vi "Read Database.vi"(8 "error in (no error)":errorcluster, 11 "Column Parent in":refnum<class "Column Parent.lvclass">) -> (0 "error out":errorcluster, 2 "Database":refnum<class "Database Interface.lvclass">, 3 "Column Parent out":refnum<class "Column Parent.lvclass">)   [LabVIEW 2020, in "Basic Columns.lvlib" / "Column Parent.lvclass"]
uses:
  Column Parent.lvclass
  Database Libraries/Database Interfaces/Database Interface Class/Database Interface.lvclass
  Column Interface/Column Configuration Interface Class/Column Configuration.lvclass
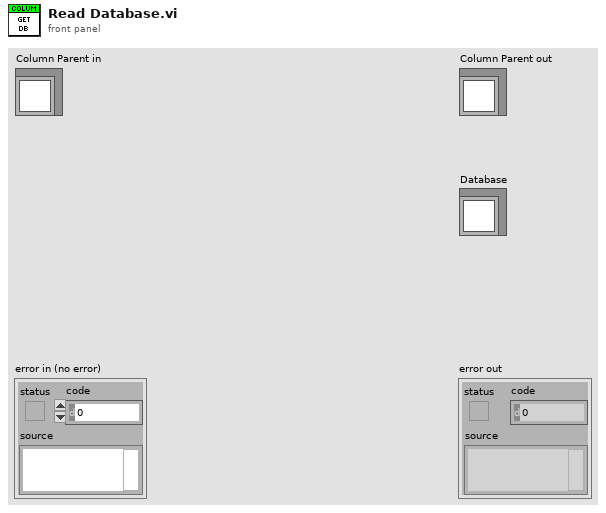
[diagram p1: front panel]
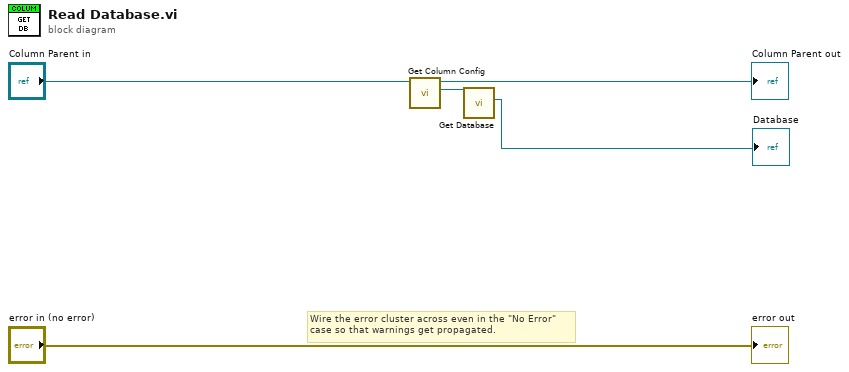
[diagram p0: block diagram]
diagram:
  # "Wire the error cluster across even in the \"No Error\"\ncase so that warnings get propagated."
  n1 = call-dynamic "Get Column Config.vi"("Column Parent in"="Column Parent in") -> ("Column Configuration"=w1:refnum<class "Column Configuration.lvclass">, "Column Parent out"=→"Column Parent out":refnum<class "Column Parent.lvclass">)  [unwired: 8 in, 1 out]
  n2 = call-dynamic "Get Database.vi"("Column Configuration in"=w1) -> ("Database"=→"Database":refnum<class "Database Interface.lvclass">)  [unwired: 8 in, 2 out]
  "error out" <- "error in (no error)"
